vi "OnResize2.vi"(0 "XRef":T17, 1 "Bounds":T15, 2 "Mouse Mods":T13, 3 "State In":T1) -> (14 "Reply":T11, 15 "Fatal Error Out":T10, 16 "State Out":T1)   [LabVIEW 2020, in "FlexBlock.xnode"]
uses:
  FlexBlock.xnode
  <vilib>/XNodeSupport/XNodeXNodeRef.ctl
  <vilib>/XNodeSupport/XNodeRect32.ctl
  <vilib>/XNodeSupport/XNodeInt.ctl
  <vilib>/XNodeSupport/XNodeMouseMods.ctl
  <vilib>/XNodeSupport/XNodeBool.ctl
  State.ctl
  FlexBlocks/Type Descriptor.ctl
  FlexBlocks/Terminal Direction.ctl
  FlexBlocks/Value Mode.ctl
  FlexBlocks/Terminal State.ctl
  FlexBlocks/Special Terminal.ctl
  FlexBlocks/Errors.ctl
  <vilib>/picture/picture.llb/imagedata.ctl
  FlexBlocks/Calculated Sizes.ctl
  <vilib>/XNodeSupport/XNodeStringArray.ctl
  <vilib>/XNodeSupport/XNodeString.ctl
  <vilib>/XNodeSupport/XNodeErrorCluster.ctl
  <vilib>/XNodeSupport/NI_XNodeSupport.lvlib
  FlexBlocks/FlexBlocks.lvlib
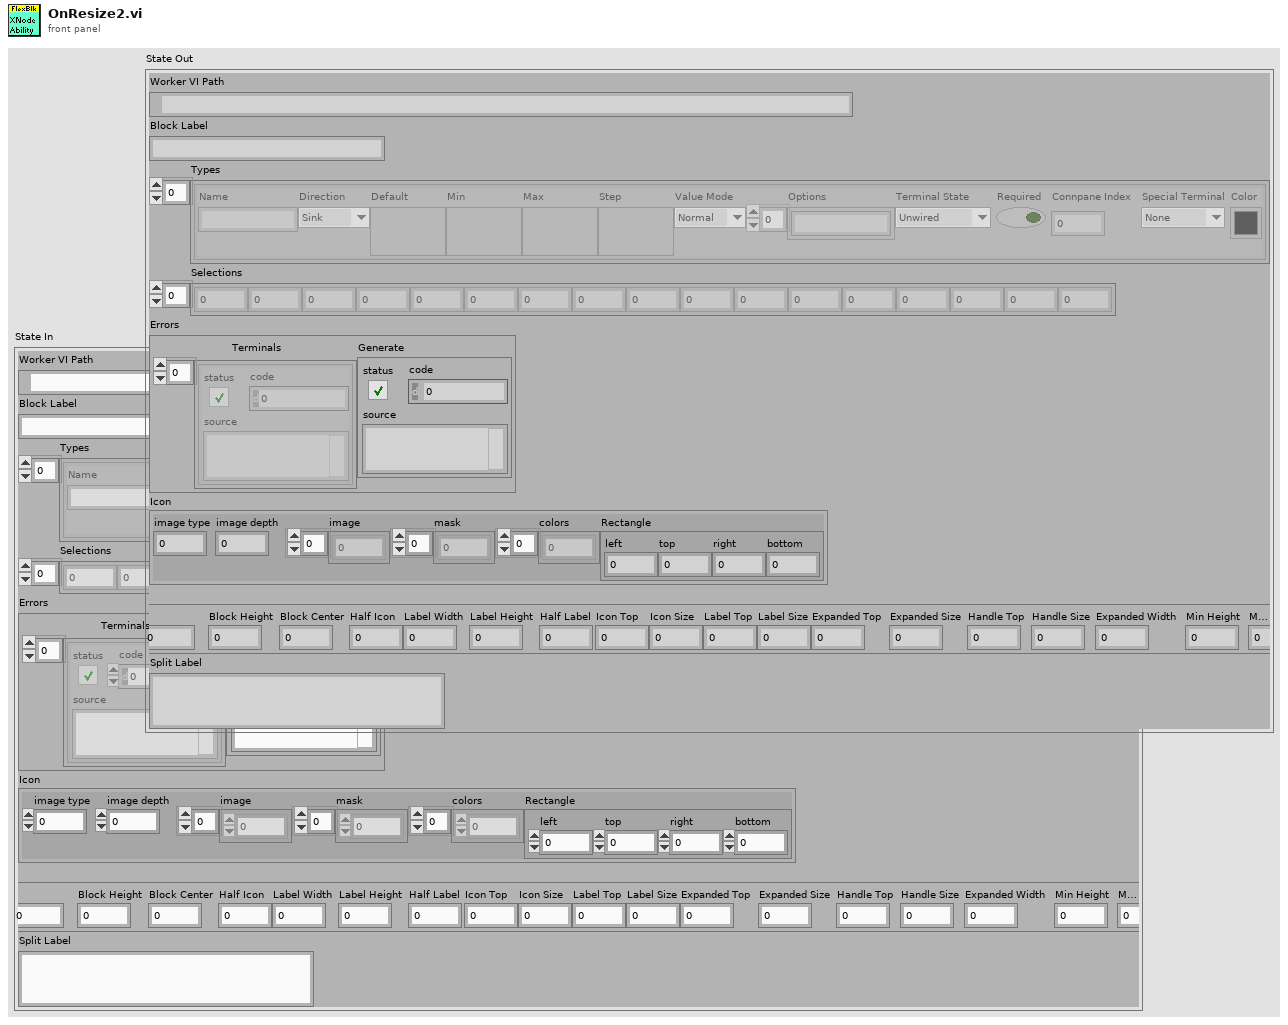
[diagram p1: front panel]
types:
  T1 = typedef "FlexBlock.xnode/State.ctl" = cluster{"Worker VI Path":path, "Block Label":string, "Types":T2[], "Selections":i32[], "Errors":T7, "Icon":T8, "Calcd Sizes":T9, "Split Label":string}
  T2 = typedef "FlexBlocks.lvlib/Type Descriptor.ctl" = cluster{"Name":string, "Direction":T3, "Default":variant, "Min":variant, "Max":variant, "Step":variant, "Value Mode":T4, "Options":string[], "Terminal State":T5, "Required":bool, "Connpane Index":i32, "Special Terminal":T6, "Color":u32}
  T3 = typedef "FlexBlocks.lvlib/Terminal Direction.ctl" = enum16{"Sink", "Source"}
  T4 = typedef "FlexBlocks.lvlib/Value Mode.ctl" = enum16{"Normal", "Range", "Select"}
  T5 = typedef "FlexBlocks.lvlib/Terminal State.ctl" = enum16{"Unwired", "BadType", "BadRef", "Channel", "Value", "Control Ref"}
  T6 = typedef "FlexBlocks.lvlib/Special Terminal.ctl" = enum16{"None", "Action", "Init", "Tag", "State in", "State out", "Error"}
  T7 = typedef "FlexBlocks.lvlib/Errors.ctl" = cluster{"Terminals":errorcluster[], "Generate":errorcluster}
  T8 = typedef "imagedata.ctl" = cluster{"image type":i32, "image depth":i32, "image":u8[], "mask":u8[], "colors":u32[], "Rectangle":cluster{"left":i16, "top":i16, "right":i16, "bottom":i16}}
  T9 = typedef "FlexBlocks.lvlib/Calculated Sizes.ctl" = cluster{"Text Width":i32, "Text Height":i32, "Half Text":i32, "Block Width":i32, "Block Height":i32, "Block Center":i32, "Half Icon":i32, "Label Width":i32, "Label Height":i32, "Half Label":i32, "Icon Top":i32, "Icon Size":i32, "Label Top":i32, "Label Size":i32, "Expanded Top":i32, "Expanded Size":i32, "Handle Top":i32, "Handle Size":i32, "Expanded Width":i32, "Min Height":i32, "Max Height":i32}
  T10 = typedef "NI_XNodeSupport.lvlib/XNodeErrorCluster.ctl" = errorcluster
  T11 = typedef "NI_XNodeSupport.lvlib/XNodeStringArray.ctl" = T12[]
  T12 = typedef "NI_XNodeSupport.lvlib/XNodeString.ctl" = string
  T13 = typedef "NI_XNodeSupport.lvlib/XNodeMouseMods.ctl" = cluster{"Shift?":T14, "Menu?":T14, "Alt?":T14}
  T14 = typedef "NI_XNodeSupport.lvlib/XNodeBool.ctl" = bool
  T15 = typedef "NI_XNodeSupport.lvlib/XNodeRect32.ctl" = cluster{"Left":T16, "Top":T16, "Right":T16, "Bottom":T16}
  T16 = typedef "NI_XNodeSupport.lvlib/XNodeInt.ctl" = i32
  T17 = typedef "NI_XNodeSupport.lvlib/XNodeXNodeRef.ctl" = refnum<vi>
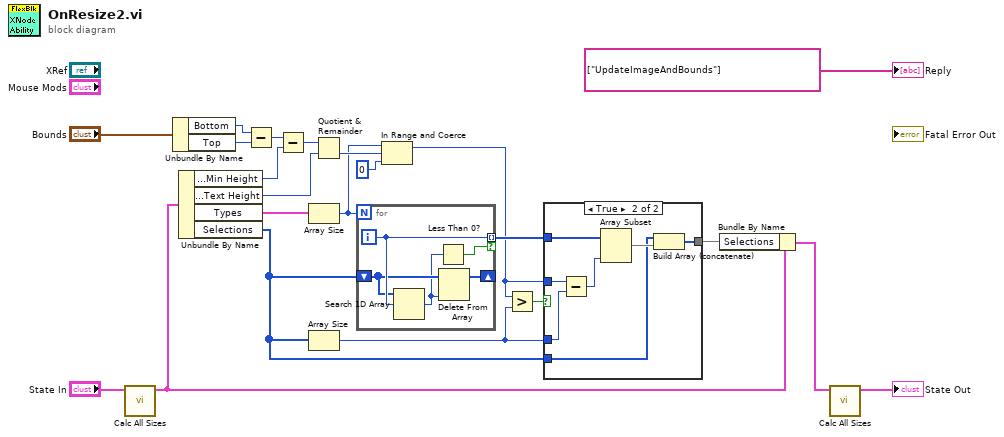
[diagram p0: block diagram]
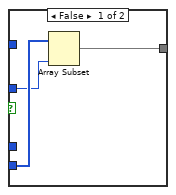
[diagram p2: hidden frame]
diagram:
  n1 = call "Calc All Sizes.vi"("State In"="State In") -> ("State"=w1:T1)  [unwired: 10 in]
  n2 = Unbundle By Name("Bounds") -> ("Bottom"=w19:T16, "Top"=w20:T16)
  n3 = Unbundle By Name(w1) -> ("Calcd Sizes.Min Height"=w17:i32, "Calcd Sizes.Text Height"=w15:i32, "Types"=w12:T2[], "Selections"=w6:i32[])
  n4 = Subtract(x=w19, y=w20) -> (x-y=w18:T16)
  n5 = Subtract(x=w18, y=w17) -> (x-y=w16:T16)
  n6 = Array Size(array=w12) -> (size(s)=w11:i32)
  n7 = Array Size(array=w6) -> (size(s)=w7:i32)
  n8 = Quotient & Remainder(x=w16, y=w15) -> (floor(x/y)=w14:T16)  [unwired: 1 out]
  n9 = for {
    N: w11 -> [_]
    shift-right: [w25] -> _
    shift-left: w6 -> [w26]
    tunnel: [w27] -> w10 mode=indexing if=w23
    i -> [w27]
    n10 = Search 1D Array(1D array=w26, element=w27) -> (index of element=w24:i32)  [unwired: 1 in]
    n11 = Less Than 0?(x=w24) -> (x < 0?=w23:bool)
    n12 = Delete From Array(array=w26, index=w24) -> (array with subset deleted=w25:i32[])  [unwired: 1 in, 1 out]
  }
  n13 = In Range and Coerce(upper limit=w11, x=w14, lower limit=T16 0) -> (coerced(x)=w8:T16)  [unwired: 1 out]
  n14 = Greater?(x=w8, y=w7) -> (0:w9:bool)
  n15 = case shown="True" w9 {
    tunnel: w10 -> [_ w35]
    tunnel: w8 -> [w29 w37]
    tunnel: w7 -> [_ w36]
    tunnel: w6 -> [w30 w32]
    tunnel: [w28 w31] -> w5
    frame False {
      n16 = Array Subset(array=w30, length=w29) -> (w28:i32[])  [unwired: 1 in]
    }
    frame True {
      n17 = Subtract(x=w37, y=w36) -> (x-y=w34:T16)
      n18 = Array Subset(array=w35, length=w34) -> (w33:i32[])  [unwired: 1 in]
      n19 = Build Array (concatenate)(w32, w33) -> (w31:i32[])
    }
  }
  n20 = Bundle By Name(cluster=w1, "Selections"=w5) -> (w4:T1)
  n21 = call "Calc All Sizes.vi"("State In"=w4) -> ("State"=→"State Out":T1)  [unwired: 10 in]
  "Reply" <- T11 ["UpdateImageAndBounds"] ("Reply")
